vi "Delete Program.vi"(8 "Error In":errorcluster, 10 "Program In":T2, 11 "Device ID":T1) -> (0 "Error Out":errorcluster)   [LabVIEW 2012]
doc: "Deletes a program."
uses:
  Non-User VIs/Controls/Program Handle.ctl
  Non-User VIs/Controls/Device ID.ctl
  Non-User VIs/Error Checking/Add Error Functional Global.vi
  OpenCLV x64.lvlib
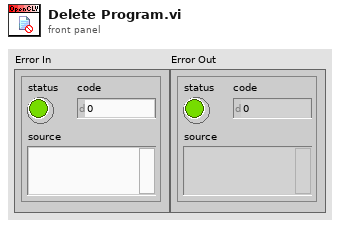
[diagram p1: front panel]
types:
  T1 = typedef "OpenCLV x64.lvlib/Device ID.ctl" = u64
  T2 = typedef "OpenCLV x64.lvlib/Program Handle.ctl" = u64
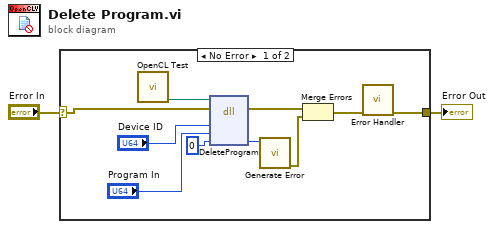
[diagram p0: block diagram]
diagram:
  n1 = case shown="No Error" "Error In" {
    selector: "Error In" -> [w3 w13]
    tunnel: [w7 w13] -> w1
    frame No Error {
      n2 = call "OpenCL Test.vi"() -> ("DLL To Use"=w8:path)  [unwired: 11 in]
      n3 = dll-call lib="C:/Users/bme-amcelroy-la/Desktop/OpenCLV/trunk/OpenCLV_x64_1.0/OpenCLV_x64.dll" fn="DeleteProgram"(path in=w8, error in=w3, "Labview Device"="Device ID", "Program Handle"="Program In", "Error"=0) -> (error out=w4:errorcluster, "Error"=w10:i32)  [unwired: 4 in, 1 out]
      n4 = call "Generate Error.vi"("Error"=w10) -> ("error out"=w6:errorcluster)  [unwired: 10 in]
      n5 = Merge Errors(w4, w6) -> (w5:errorcluster)
      n6 = call-poly "Error Handler.vi"("Error In"=w5) -> ("Error Out"=w7:errorcluster)  [unwired: 10 in]
    }
    frame Error {
    }
  }
  "Error Out" <- w1
